vi "SaveDataFile.vi"(0 "Data Array":dbl[][](array[numeric]), 1 "Temperature":dbl, 3 "Humidity":dbl, 11 "Error In":errorcluster, 12 "Array Titles":string, 13 "Strip Segment":string) -> (4 "Filename OUT":string, 6 "Pathname OUT":string, 10 "Path + Filename OUT":string, 15 "Error Out":errorcluster)   [LabVIEW 2019]
uses:
  globals/QC_RunInformation.vi
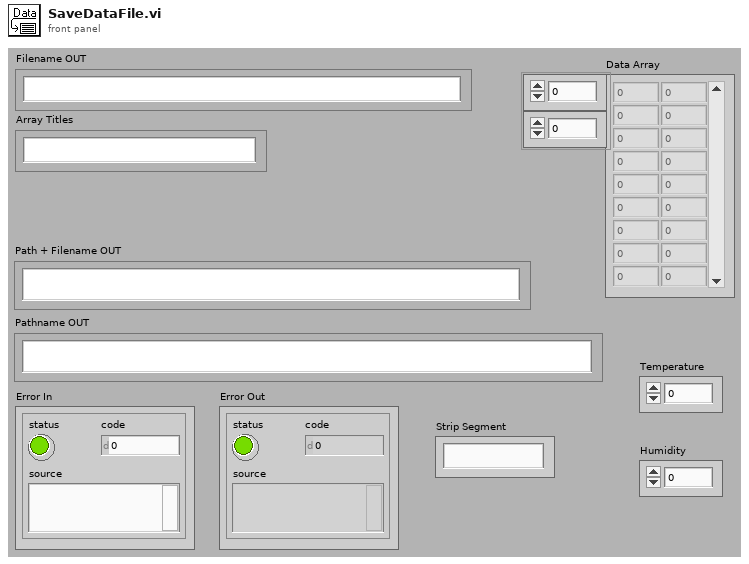
[diagram p1: front panel]
types:
  T1 = enum16{"open", "open or create", "create or replace", "create"}
  T2 = cluster{"Sensor Serial No.:":string, "Wafer Serial No.:":string, "Batch:":string, "Manufacturer:":string, "Device Category:":string, "Database Serial No.:":string, "Date Initiated:":string, "Time Initiated:":string, "Test":string, "Instruments used:":string, "Probeplan used:":string, "End of Run comment:":string, "User:":string}
  T3 = cluster{"Institute":string, "Manufacturers":string[], "Devices":string[], "Serialnumbers Lookup DB":string, "Data directory":string, "Backup & screenshot directory":string, "List of known users":string[], "Measurement switch not used":bool, "Measurement Switch":string, "DUT Switch":string}
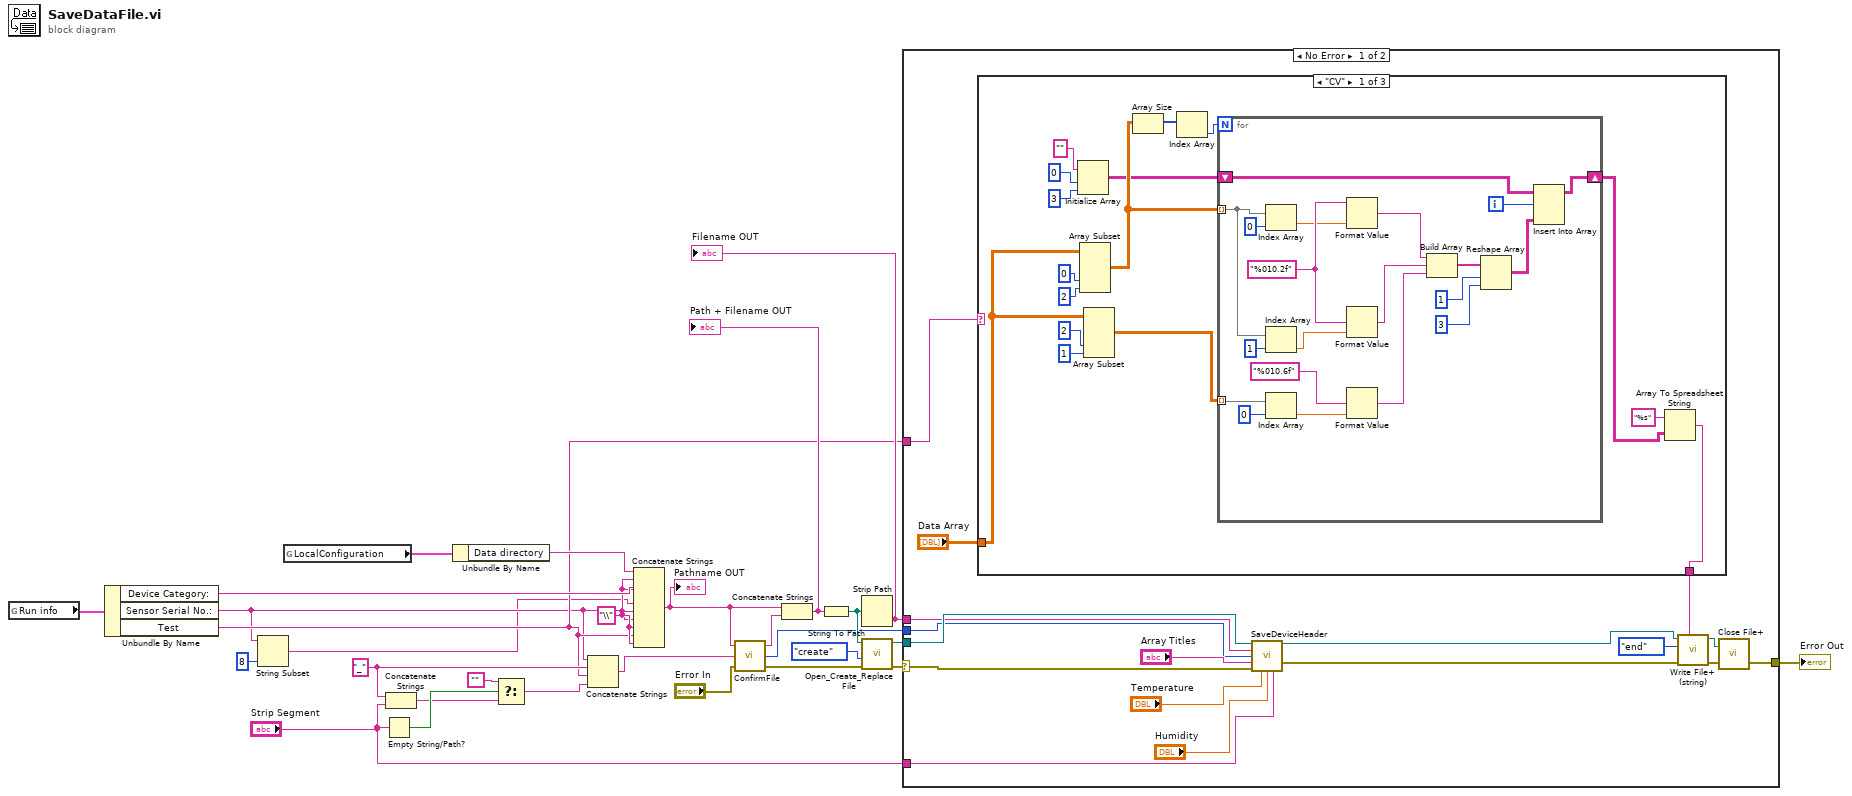
[diagram p0: block diagram]
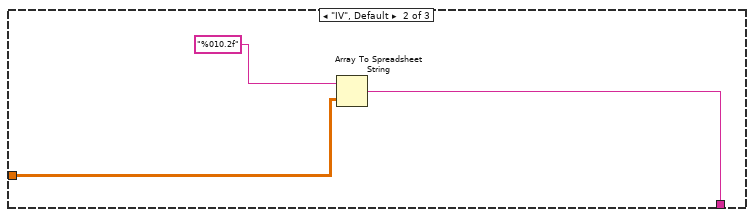
[diagram p2: hidden frame]
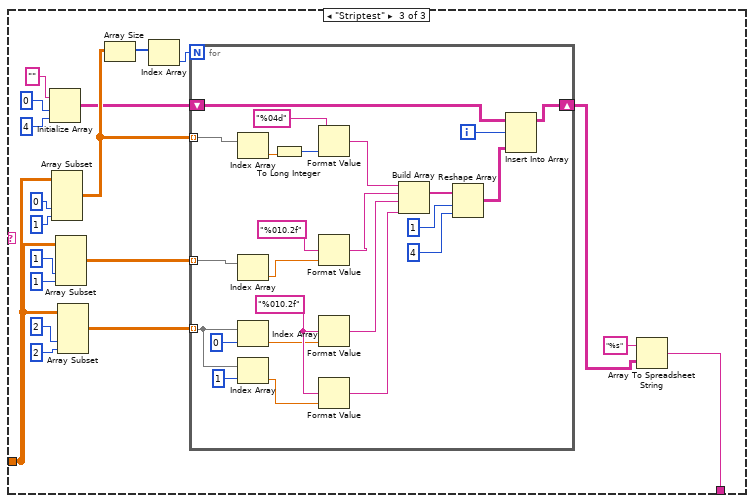
[diagram p3: hidden frame]
diagram:
  w9 = "_"
  w19 = "\\"
  n1 = global read "QC_RunInformation.vi" "Run info"() -> (w27:T2)
  n2 = Unbundle By Name(w27) -> ("Device Category:"=w25:string, "Sensor Serial No.:"=w3:string, "Test"=w4:string)
  n3 = String Subset(string=w3, length (rest)=8 ("length (rest)")) -> (substring=w1:string)  [unwired: 1 in]
  n4 = global read "QC_RunInformation.vi" "LocalConfiguration"() -> (w28:T3)
  n5 = Empty String/Path?(string/path="Strip Segment") -> (empty?=w11:bool)
  n6 = Concatenate Strings(w9, "Strip Segment") -> (w7:string)
  n7 = Unbundle By Name(w28) -> ("Data directory"=w26:string)
  n8 = Select(t="", s=w11, f=w7) -> (s? t:f=w8:string)
  n9 = Concatenate Strings(w3, w9, w4, w8) -> (w18:string)
  n10 = Concatenate Strings(w26, w19, w25, w19, w1, w19, w3, w19, w4, w19) -> (w14:string)
  "Pathname OUT" <- w14
  n11 = call "ConfirmFile.vi"("Error In"="Error In", "Filename IN"=w18, "Pathname IN"=w14) -> ("Error Out"=w15:errorcluster, "Run Number"=w6:i32, "Filename:"=w13:string)
  n12 = Concatenate Strings(w14, w13) -> (w12:string)
  "Path + Filename OUT" <- w12
  n13 = String To Path(string=w12) -> (path=w21:path)
  n14 = Strip Path(path=w21) -> (name=w22:string)  [unwired: 1 out]
  "Filename OUT" <- w22
  n15 = call <vilib>:"Open_Create_Replace File.vi"("error in (no error)"=w15, "function (open:0)"=T1."create", "file path"=w21) -> ("error out"=w20:errorcluster, "refnum"=w23:refnum<file>)  [unwired: 5 in, 2 out]
  n16 = case shown="No Error" w20 {
    selector: w20 -> [w45 w128]
    tunnel: w23 -> [w39 _]
    tunnel: w22 -> [w38 _]
    tunnel: [w36 w128] -> w17
    tunnel: w6 -> [w32 _]
    tunnel: "Strip Segment" -> [w31 _]
    tunnel: w4 -> [w29 _]
    frame No Error {
      n17 = case shown="\"CV\"" w29 {
        tunnel: [w46 w84 w87] -> w44
        tunnel: "Data Array" -> [w48 w83 w98]
        frame "CV" {
          n18 = Initialize Array("", 0 ("dimension size"), 3 ("dimension size")) -> (w51:string[][])
          n19 = Array Subset(array=w48, index (col)=0 ("index"), length (col)=2 ("length")) -> (w54:dbl[][])  [unwired: 2 in]
          n20 = Array Subset(array=w48, index (col)=2 ("index"), length (col)=1 ("length")) -> (w47:dbl[][])  [unwired: 2 in]
          n21 = Array Size(array=w54) -> (size(s)=w53:i32[])
          n22 = Index Array(array=w53) -> (element=w52:i32)  [unwired: 1 in]
          n23 = for {
            N: w52 -> [_]
            tunnel: w47 -> [w77] mode=indexing
            tunnel: w54 -> [w66] mode=indexing
            shift-right: [w80] -> w49
            shift-left: w51 -> [w79]
            i -> [w81]
            w63 = "%010.2f" ("format string")
            n24 = Index Array(array=w66, index=0) -> (element=w62:dbl)
            n25 = Index Array(array=w66, index=1) -> (element=w76:dbl)
            n26 = Index Array(array=w77, index=0) -> (element=w74:dbl)
            n27 = Format Value(string ("")=w63, value (0)=w62) -> (output string=w73:string)  [unwired: 1 in]
            n28 = Format Value(format string=w63, value (0)=w76) -> (output string=w72:string)  [unwired: 1 in]
            n29 = Format Value(format string="%010.6f", value (0)=w74) -> (output string=w71:string)  [unwired: 1 in]
            n30 = Build Array(w73, w72, w71) -> (w70:string[])
            n31 = Reshape Array(w70, 1 ("dimension size"), 3 ("dimension size")) -> (w67:string[][])
            n32 = Insert Into Array(array=w79, index (row)=w81, new element=w67) -> (w80:string[][])  [unwired: 1 in]
          }
          n33 = Array To Spreadsheet String(array=w49, 3:"%s" ("format string")) -> (spreadsheet string=w46:string)  [unwired: 1 in]
        }
        frame "IV", Default {
          n34 = Array To Spreadsheet String(array=w83, 3:"%010.2f") -> (spreadsheet string=w84:string)  [unwired: 1 in]
        }
        frame "Striptest" {
          n35 = Initialize Array("", 0 ("dimension size"), 4 ("dimension size")) -> (w88:string[][])
          n36 = Array Subset(array=w98, index (col)=0 ("index"), length (col)=1 ("length")) -> (w91:dbl[][])  [unwired: 2 in]
          n37 = Array Subset(array=w98, index (col)=1 ("index"), length (col)=1 ("length")) -> (w93:dbl[][])  [unwired: 2 in]
          n38 = Array Subset(array=w98, index (col)=2 ("index"), length (col)=2 ("length")) -> (w92:dbl[][])  [unwired: 2 in]
          n39 = Array Size(array=w91) -> (size(s)=w90:i32[])
          n40 = Index Array(array=w90) -> (element=w89:i32)  [unwired: 1 in]
          n41 = for {
            N: w89 -> [_]
            tunnel: w93 -> [w120] mode=indexing
            tunnel: w92 -> [w123] mode=indexing
            tunnel: w91 -> [w121] mode=indexing
            shift-right: [w126] -> w85
            shift-left: w88 -> [w125]
            i -> [w127]
            w114 = "%010.2f" ("format string")
            n42 = Index Array(array=w121) -> (element=w118:dbl)  [unwired: 1 in]
            n43 = Index Array(array=w120) -> (element=w116:dbl)  [unwired: 1 in]
            n44 = Index Array(array=w123, index=0) -> (element=w113:dbl)
            n45 = Index Array(array=w123, index=1) -> (element=w112:dbl)
            n46 = To Long Integer(number=w118) -> (32bit integer=w119:i32)
            n47 = Format Value(format string="%04d", value (0)=w119) -> (output string=w111:string)  [unwired: 1 in]
            n48 = Format Value(format string="%010.2f", value (0)=w116) -> (output string=w110:string)  [unwired: 1 in]
            n49 = Format Value(format string=w114, value (0)=w113) -> (output string=w109:string)  [unwired: 1 in]
            n50 = Format Value(format string=w114, value (0)=w112) -> (output string=w108:string)  [unwired: 1 in]
            n51 = Build Array(w111, w110, w109, w108) -> (w107:string[])
            n52 = Reshape Array(w107, 1 ("dimension size"), 4 ("dimension size")) -> (w104:string[][])
            n53 = Insert Into Array(array=w125, index (row)=w127, new element=w104) -> (w126:string[][])  [unwired: 1 in]
          }
          n54 = Array To Spreadsheet String(array=w85, 3:"%s" ("format string")) -> (spreadsheet string=w87:string)  [unwired: 1 in]
        }
      }
      n55 = call "SaveDeviceHeader.vi"("File Refnum in"=w39, "Filename"=w38, "Run Number"=w32, "Array Titles"="Array Titles", "error in (no error)"=w45, "Temperature"="Temperature", "Humidity"="Humidity", "Strip Structure"=w31) -> ("File Refnum out"=w40:refnum<file>, "error out"=w33:errorcluster)  [unwired: 5 in, 1 out]
      n56 = call <vilib>:"Write File+ (string).vi"("string"=w44, "error in (no error)"=w33, "pos mode (rel. to end:1)"=enum16{"start", "end", "current"}."end", "refnum"=w40) -> ("error out"=w43:errorcluster, "dup refnum"=w41:refnum<file>)  [unwired: 3 in, 1 out]
      n57 = call <vilib>:"Close File+.vi"("error in (no error)"=w43, "refnum"=w41) -> ("error out"=w36:errorcluster)  [unwired: 3 in, 2 out]
    }
    frame Error {
    }
  }
  "Error Out" <- w17
